vi "Comp_16_Elements.vi"(10 "Array":u16[](array[numeric])=[0, 0, 0, 0, 0, 0, 0, 0, 0, 0, 0, 0, 0, 0, 0, 0], 11 "CompVal":u16) -> (3 "result":bool)   [LabVIEW 2016]
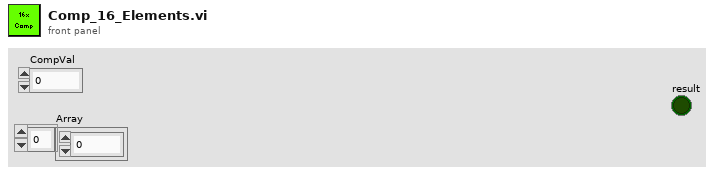
[diagram p1: front panel]
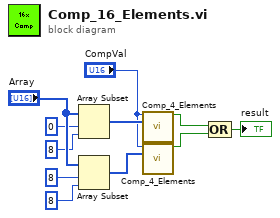
[diagram p0: block diagram]
diagram:
  n1 = Array Subset(array="Array", index=0, length=8 ("index")) -> (w6:u16[])
  n2 = Array Subset(array="Array", index=8, length=8 ("index")) -> (w10:u16[])
  n3 = call "Comp_4_Elements.vi"("CompVal"="CompVal", "Array"=w6) -> ("result"=w3:bool)  [unwired: 13 in]
  n4 = call "Comp_4_Elements.vi"("CompVal"="CompVal", "Array"=w10) -> ("result"=w4:bool)  [unwired: 13 in]
  n5 = Compound Arithmetic op=OR(w3, w4) -> (→"result":bool)
